vi "Vision - Set Array Size.vi"(4 "Panel Bounds":T2, 5 "Thumbnail?":enum16{"CAT", "RCA_L", "RCA_R"}(ring), 6 "Panel Size":T1, 7 "Initialise?":bool, 8 "error in (no error)":errorcluster, 9 "Draw Area Size":T1, 10 "Rectangle":T3, 11 "Image ThumbNails":refnum<vi>) -> (0 "error out":errorcluster)   [LabVIEW 2024]
uses:
  <vilib>/Utility/miscctls.llb/LVBoundsTypeDef.ctl
  <vilib>/Utility/miscctls.llb/LVRectTypeDef.ctl
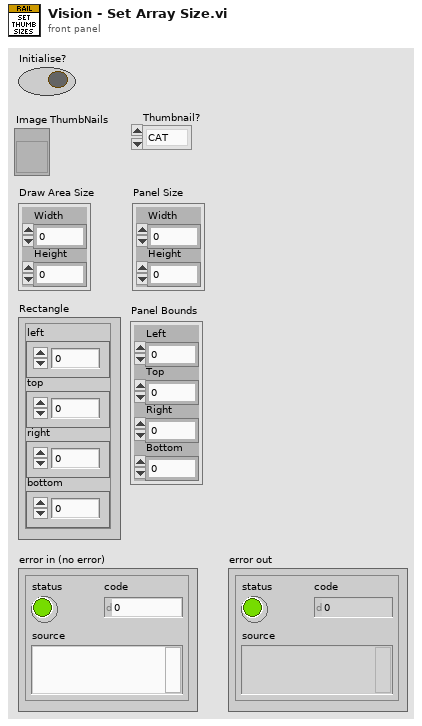
[diagram p1: front panel]
types:
  T1 = typedef "LVBoundsTypeDef.ctl" = cluster{"Width":u32, "Height":u32}
  T2 = typedef "LVRectTypeDef.ctl" = cluster{"Left":i16, "Top":i16, "Right":i16, "Bottom":i16}
  T3 = cluster{"left":i16, "top":i16, "right":i16, "bottom":i16}
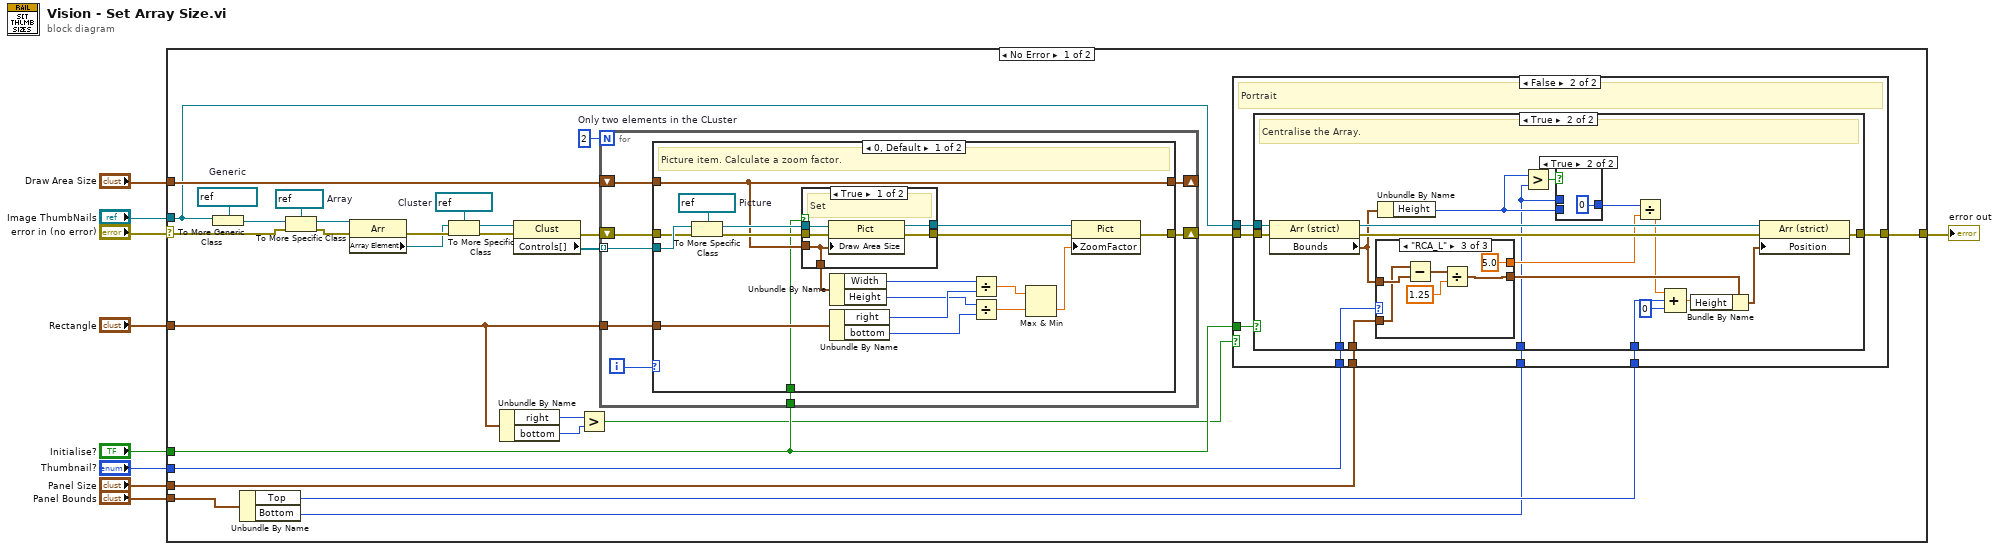
[diagram p0: block diagram]
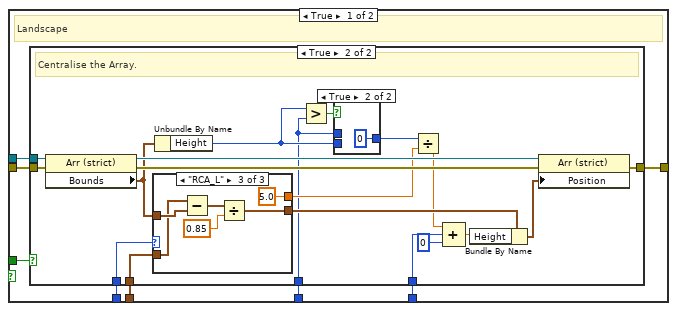
[diagram p2: hidden frame]
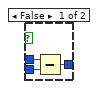
[diagram p4: hidden frame]
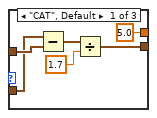
[diagram p5: hidden frame]
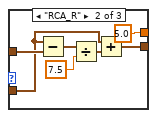
[diagram p6: hidden frame]
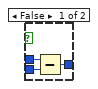
[diagram p8: hidden frame]
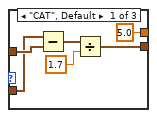
[diagram p9: hidden frame]
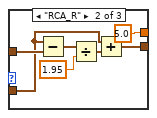
[diagram p10: hidden frame]
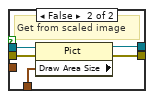
[diagram p11: hidden frame]
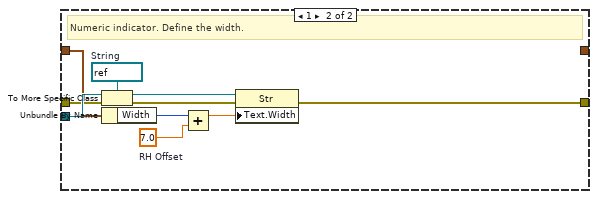
[diagram p12: hidden frame]
diagram:
  n1 = case shown="No Error" "error in (no error)" {
    selector: "error in (no error)" -> [w23 w187]
    tunnel: "Image ThumbNails" -> [w22 _]
    tunnel: "Draw Area Size" -> [w24 _]
    tunnel: [w20 w187] -> w6
    tunnel: "Initialise?" -> [w16 _]
    tunnel: "Rectangle" -> [w13 _]
    tunnel: "Panel Size" -> [w19 _]
    tunnel: "Panel Bounds" -> [w18 _]
    tunnel: "Thumbnail?" -> [w15 _]
    frame No Error {
      w25 = 2  # Only two elements in the CLuster
      w30 = refnum<vi> refnum  # Cluster
      w35 = refnum<vi> refnum  # Array
      w37 = refnum<vi> refnum  # Generic
      n2 = To More Generic Class(target class=w37, reference=w22) -> (generic class reference=w36:refnum<vi>)
      n3 = Unbundle By Name(w18) -> ("Top"=w17:i16, "Bottom"=w14:i16)
      n4 = To More Specific Class(target class=w35, reference=w36, error in=w23) -> (specific class reference=w34:refnum<vi>, error out=w33:errorcluster)
      n5 = property on="Property Node" class="Arr"(reference=w34, error in=w33) -> (error out=w32:errorcluster, "Array Element"=w31:refnum<vi>)  [unwired: 1 out]
      n6 = To More Specific Class(target class=w30, reference=w31, error in=w32) -> (specific class reference=w29:refnum<vi>, error out=w28:errorcluster)
      n7 = Unbundle By Name(w13) -> ("right"=w12:i16, "bottom"=w11:i16)
      n8 = property on="Property Node" class="Clust"(reference=w29, error in=w28) -> (error out=w27:errorcluster, "Controls[]"=w26:refnum<vi>[])  [unwired: 1 out]
      n9 = Greater?(x=w12, y=w11) -> (0:w10:bool)
      n10 = for {
        N: w25 -> [_]
        tunnel: w26 -> [w146] mode=indexing
        shift-right: [w143] -> w21
        shift-left: w27 -> [w145]
        tunnel: w13 -> [w142]
        shift-right: [w141] -> _
        shift-left: w24 -> [w144]
        tunnel: w16 -> [w140]
        i -> [w147]
        n11 = case shown="0, Default" w147 {
          tunnel: w146 -> [w165 w185]
          tunnel: w145 -> [w164 w184]
          tunnel: w144 -> [w150 w180]
          tunnel: [w152 w181] -> w143
          tunnel: w142 -> [w151 _]
          tunnel: [w150 _] -> w141
          tunnel: w140 -> [w149 _]
          frame 0, Default {
            w166 = refnum<vi> refnum  # Picture
            # "Picture item. Calculate a zoom factor."
            n12 = To More Specific Class(target class=w166, reference=w165, error in=w164) -> (specific class reference=w163:refnum<vi>, error out=w162:errorcluster)
            n13 = case shown="True" w149 {
              tunnel: w163 -> [w171 w176]
              tunnel: w162 -> [w170 w175]
              tunnel: [w169 w174] -> w154
              tunnel: [w168 w173] -> w153
              tunnel: w150 -> [w167 _]
              tunnel: [w167 w172] -> w148
              frame True {
                # "Set"
                n14 = property on="Property Node" class="Pict"(reference=w171, error in=w170, "Draw Area Size"=w167) -> (reference out=w168:refnum<vi>, error out=w169:errorcluster)
              }
              frame False {
                # "Get from scaled image"
                n15 = property on="Property Node" class="Pict"(reference=w176, error in=w175) -> (reference out=w173:refnum<vi>, error out=w174:errorcluster, "Draw Area Size"=w172:T1)
              }
            }
            n16 = Unbundle By Name(w148) -> ("Width"=w155:u32, "Height"=w156:u32)
            n17 = Unbundle By Name(w151) -> ("right"=w160:i16, "bottom"=w161:i16)
            n18 = Divide(x=w155, y=w160) -> (x/y=w157:dbl)
            n19 = Divide(x=w156, y=w161) -> (x/y=w158:dbl)
            n20 = Max & Min(x=w157, y=w158) -> (min(x,y)=w159:dbl)  [unwired: 1 out]
            n21 = property on="Property Node" class="Pict"(reference=w153, error in=w154, "ZoomFactor"=w159) -> (error out=w152:errorcluster)  [unwired: 1 out]
          }
          frame 1 {
            w177 = 7.0  # RH Offset
            w186 = refnum<vi> refnum  # String
            # "Numeric indicator. Define the width."
            n22 = To More Specific Class(target class=w186, reference=w185, error in=w184) -> (specific class reference=w183:refnum<vi>, error out=w182:errorcluster)
            n23 = Unbundle By Name(w180) -> ("Width"=w179:u32)
            n24 = Add(x=w179, y=w177) -> (x+y=w178:dbl)
            n25 = property on="Property Node" class="Str"(reference=w183, error in=w182, "Text.Width"=w178) -> (error out=w181:errorcluster)  [unwired: 1 out]
          }
        }
      }
      n26 = case shown="False" w10 {
        tunnel: w22 -> [w45 w96]
        tunnel: w21 -> [w44 w95]
        tunnel: [w43 w94] -> w20
        tunnel: w19 -> [w42 w93]
        tunnel: w17 -> [w41 w92]
        tunnel: w16 -> [w40 w91]
        tunnel: w15 -> [w39 w90]
        tunnel: w14 -> [w38 w89]
        frame True {
          # "Landscape"
          n27 = case shown="True" w40 {
            tunnel: w45 -> [_ w61]
            tunnel: w44 -> [w46 w60]
            tunnel: [w46 w59] -> w43
            tunnel: w42 -> [_ w57]
            tunnel: w41 -> [_ w56]
            tunnel: w39 -> [_ w54]
            tunnel: w38 -> [_ w48]
            frame False {
            }
            frame True {
              # "Centralise the Array."
              n28 = property on="Property Node" class="Arr (strict)"(reference=w61, error in=w60) -> (reference out=w58:refnum<vi>, error out=w65:errorcluster, "Bounds"=w53:T1)
              n29 = case shown="\"RCA_L\"" w54 {
                tunnel: w53 -> [w75 w78 w88]
                tunnel: [w73 w79 w86] -> w64
                tunnel: w57 -> [w72 w77 w85]
                tunnel: [5.0 ("y") 5.0 ("y") 5.0 ("y")] -> w50
                frame "CAT", Default {
                  n30 = Subtract(x=w72, y=w75) -> (x-y=w74:T1)
                  n31 = Divide(x=w74, y=1.7 ("Numeric")) -> (x/y=w73:cluster{"Width":dbl, "Height":dbl})
                }
                frame "RCA_R" {
                  n32 = Subtract(x=w77, y=w78) -> (x-y=w82:T1)
                  n33 = Divide(x=w82, y=7.5 ("Numeric")) -> (x/y=w81:cluster{"Width":dbl, "Height":dbl})
                  n34 = Add(x=w77, y=w81) -> (x+y=w79:cluster{"Width":dbl, "Height":dbl})
                }
                frame "RCA_L" {
                  n35 = Subtract(x=w85, y=w88) -> (x-y=w87:T1)
                  n36 = Divide(x=w87, y=0.85 ("Numeric")) -> (x/y=w86:cluster{"Width":dbl, "Height":dbl})
                }
              }
              n37 = Unbundle By Name(w53) -> ("Height"=w49:u32)
              n38 = Greater?(x=w49, y=w48) -> (0:w47:bool)
              n39 = case shown="True" w47 {
                tunnel: [w68 u32 0] -> w52
                tunnel: w49 -> [w67 _]
                tunnel: w48 -> [w66 _]
                frame False {
                  n40 = Subtract(x=w66, y=w67) -> (x-y=w68:u32)
                }
                frame True {
                }
              }
              n41 = Divide(x=w52, y=w50) -> (x/y=w51:dbl)
              n42 = Compound Arithmetic op=ADD(w51, w56, i16 0 ("y")) -> (w63:dbl)
              n43 = Bundle By Name(cluster=w64, "Height"=w63) -> (w62:cluster{"Width":dbl, "Height":dbl})
              n44 = property on="Property Node" class="Arr (strict)"(reference=w58, error in=w65, "Position"=w62) -> (error out=w59:errorcluster)  [unwired: 1 out]
            }
          }
        }
        frame False {
          # "Portrait"
          n45 = case shown="True" w91 {
            tunnel: w96 -> [_ w112]
            tunnel: w95 -> [w97 w111]
            tunnel: [w97 w110] -> w94
            tunnel: w93 -> [_ w108]
            tunnel: w92 -> [_ w107]
            tunnel: w90 -> [_ w105]
            tunnel: w89 -> [_ w99]
            frame False {
            }
            frame True {
              # "Centralise the Array."
              n46 = property on="Property Node" class="Arr (strict)"(reference=w112, error in=w111) -> (reference out=w109:refnum<vi>, error out=w116:errorcluster, "Bounds"=w104:T1)
              n47 = case shown="\"RCA_L\"" w105 {
                tunnel: w104 -> [w126 w129 w139]
                tunnel: [w124 w130 w134] -> w115
                tunnel: w108 -> [w123 w128 w138]
                tunnel: [5.0 ("y") 5.0 ("y") 5.0 ("y")] -> w101
                frame "CAT", Default {
                  n48 = Subtract(x=w123, y=w126) -> (x-y=w125:T1)
                  n49 = Divide(x=w125, y=1.7 ("Numeric")) -> (x/y=w124:cluster{"Width":dbl, "Height":dbl})
                }
                frame "RCA_R" {
                  n50 = Subtract(x=w128, y=w129) -> (x-y=w133:T1)
                  n51 = Divide(x=w133, y=1.95 ("Numeric")) -> (x/y=w132:cluster{"Width":dbl, "Height":dbl})
                  n52 = Add(x=w128, y=w132) -> (x+y=w130:cluster{"Width":dbl, "Height":dbl})
                }
                frame "RCA_L" {
                  n53 = Subtract(x=w138, y=w139) -> (x-y=w135:T1)
                  n54 = Divide(x=w135, y=1.25 ("Numeric")) -> (x/y=w134:cluster{"Width":dbl, "Height":dbl})
                }
              }
              n55 = Unbundle By Name(w104) -> ("Height"=w100:u32)
              n56 = Greater?(x=w100, y=w99) -> (0:w98:bool)
              n57 = case shown="True" w98 {
                tunnel: [w119 u32 0] -> w103
                tunnel: w100 -> [w118 _]
                tunnel: w99 -> [w117 _]
                frame False {
                  n58 = Subtract(x=w117, y=w118) -> (x-y=w119:u32)
                }
                frame True {
                }
              }
              n59 = Divide(x=w103, y=w101) -> (x/y=w102:dbl)
              n60 = Compound Arithmetic op=ADD(w102, w107, i16 0 ("y")) -> (w114:dbl)
              n61 = Bundle By Name(cluster=w115, "Height"=w114) -> (w113:cluster{"Width":dbl, "Height":dbl})
              n62 = property on="Property Node" class="Arr (strict)"(reference=w109, error in=w116, "Position"=w113) -> (error out=w110:errorcluster)  [unwired: 1 out]
            }
          }
        }
      }
    }
    frame Error {
    }
  }
  "error out" <- w6
